vi "Make Joystick JSON.vi"(9 "Force":bool, 10 "Joystick prev":T1={"type"="Joystick", "device"="3", "name"="", "data"={"<init"=FALSE, ">buttons"=[], ">povs"=[], ">axes"=[], "<left_rumble"=0.0, "<right_rumble"=0.0, "<outputs"=0}}, 11 "Joystick new":T1={"type"="Joystick", "device"="3", "name"="", "data"={"<init"=FALSE, ">buttons"=[], ">povs"=[], ">axes"=[], "<left_rumble"=0.0, "<right_rumble"=0.0, "<outputs"=0}}) -> (3 "JSON delta":string)   [LabVIEW 2019]
uses:
  Joystick data proto.ctl
  Joystick proto.ctl
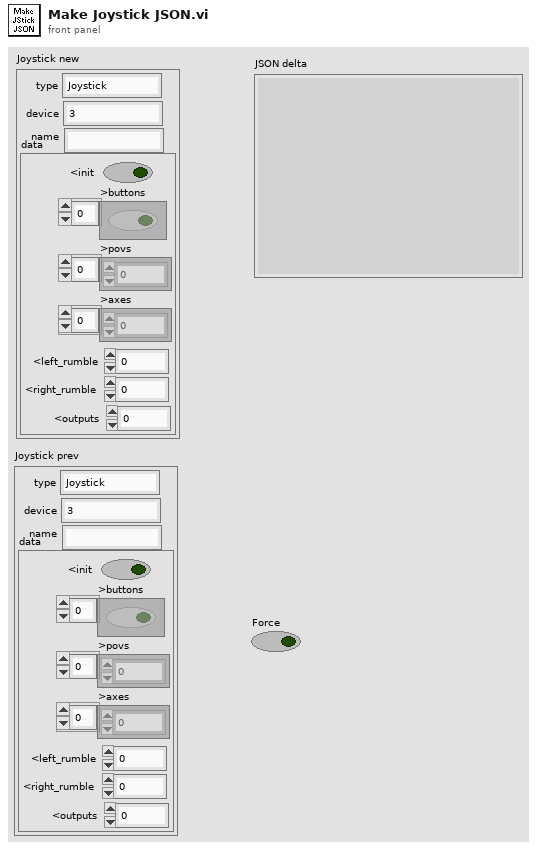
[diagram p1: front panel]
types:
  T1 = typedef "Joystick proto.ctl" = cluster{"type":string, "device":string, "name":string, "data":T2}
  T2 = typedef "Joystick data proto.ctl" = cluster{"<init":bool, ">buttons":bool[], ">povs":i32[], ">axes":i32[], "<left_rumble":dbl, "<right_rumble":dbl, "<outputs":i32}
  T3 = cluster{"type":bool, "device":bool, "name":bool, "data":cluster{"<init":bool, ">buttons":bool[], ">povs":bool[], ">axes":bool[], "<left_rumble":bool, "<right_rumble":bool, "<outputs":bool}}
  T4 = cluster{"<init":bool, ">buttons":bool[], ">povs":bool[], ">axes":bool[], "<left_rumble":bool, "<right_rumble":bool, "<outputs":bool}
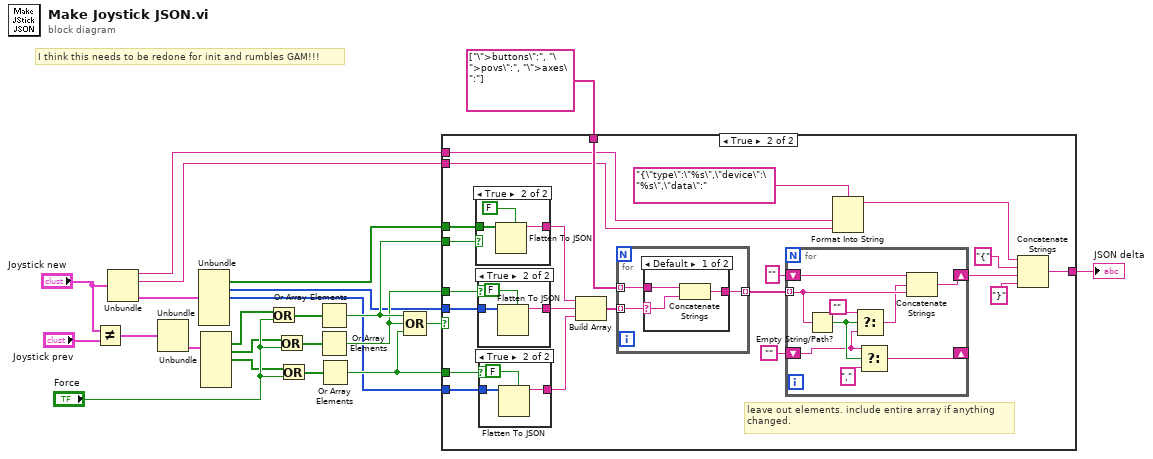
[diagram p0: block diagram]
diagram:
  # "I think this needs to be redone for init and rumbles GAM!!!"
  n1 = Not Equal?(x="Joystick new", y="Joystick prev") -> (x != y?=w7:T3)
  n2 = Unbundle("Joystick new") -> ("type"=w14:string, "device"=w15:string, "data"=w13:T2)  [unwired: 1 out]
  n3 = Unbundle(w7) -> ("data"=w12:T4)  [unwired: 3 out]
  n4 = Unbundle(w13) -> (">buttons"=w4:bool[], ">povs"=w5:i32[], ">axes"=w6:i32[])  [unwired: 4 out]
  n5 = Unbundle(w12) -> (">buttons"=w1:bool[], ">povs"=w2:bool[], ">axes"=w3:bool[])  [unwired: 4 out]
  n6 = Or(x=w1, y="Force") -> (x .or. y?=w10:bool[])
  n7 = Or(x=w2, y="Force") -> (x .or. y?=w9:bool[])
  n8 = Or(x=w3, y="Force") -> (x .or. y?=w8:bool[])
  n9 = Or Array Elements(Boolean array=w10) -> (logical OR=w19:bool)
  n10 = Or Array Elements(Boolean array=w9) -> (logical OR=w18:bool)
  n11 = Or Array Elements(Boolean array=w8) -> (logical OR=w17:bool)
  n12 = Compound Arithmetic op=OR(w19, w18, w17) -> (w16:bool)
  n13 = case shown="True" w16 {
    tunnel: w19 -> [_ w45]
    tunnel: w4 -> [_ w44]
    tunnel: w18 -> [_ w43]
    tunnel: w5 -> [_ w42]
    tunnel: w17 -> [_ w41]
    tunnel: w6 -> [_ w40]
    tunnel: string[] ["\">buttons\":", "\">povs\":", "\">axes\":"] -> [_ w36]
    tunnel: [_ w30] -> w20
    tunnel: w15 -> [_ w25]
    tunnel: w14 -> [_ w24]
    frame False {
    }
    frame True {
      # "leave out elements. include entire array if anything\nchanged."
      n14 = case shown="True" w45 {
        tunnel: w44 -> [_ w69]
        tunnel: [_ w67] -> w39
        frame False {
        }
        frame True {
          n15 = Flatten To JSON(enable LabVIEW extensions? (T)=FALSE, anything=w69) -> (JSON string=w67:string)  [unwired: 1 in, 1 out]
        }
      }
      n16 = case shown="True" w43 {
        tunnel: w42 -> [_ w66]
        tunnel: [_ w64] -> w38
        frame False {
        }
        frame True {
          n17 = Flatten To JSON(enable LabVIEW extensions? (T)=FALSE, anything=w66) -> (JSON string=w64:string)  [unwired: 1 in, 1 out]
        }
      }
      n18 = case shown="True" w41 {
        tunnel: w40 -> [_ w63]
        tunnel: [_ w61] -> w37
        frame False {
        }
        frame True {
          n19 = Flatten To JSON(enable LabVIEW extensions? (T)=FALSE, anything=w63) -> (JSON string=w61:string)  [unwired: 1 in, 1 out]
        }
      }
      n20 = Build Array(w39, w38, w37) -> (w35:string[])
      n21 = for {
        tunnel: w36 -> [w56] mode=indexing
        tunnel: w35 -> [w57] mode=indexing
        tunnel: [w55] -> w34 mode=indexing
        n22 = case shown="Default" w57 {
          selector: w57 -> [w59 _]
          tunnel: w56 -> [w60 _]
          tunnel: [w58 _] -> w55
          frame Default {
            n23 = Concatenate Strings(w60, w59) -> (w58:string)
          }
          frame "" {
          }
        }
      }
      n24 = for {
        tunnel: w34 -> [w51] mode=indexing
        shift-right: [w52] -> w33
        shift-left: "" -> [w54]
        shift-right: [w50] -> _
        shift-left: "" -> [w46]
        n25 = Empty String/Path?(string/path=w51) -> (empty?=w49:bool)
        n26 = Select(t="", s=w49, f=w46) -> (s? t:f=w48:string)
        n27 = Select(t=w46, s=w49, f=",") -> (s? t:f=w50:string)
        n28 = Concatenate Strings(w54, w48, w51) -> (w52:string)
      }
      n29 = Format Into String(format string="{\"type\":\"%s\",\"device\":\"%s\",\"data\":", w24, w25) -> (resulting string=w26:string)  [unwired: 2 in, 1 out]
      n30 = Concatenate Strings(w26, "{", w33, "}") -> (w30:string)
    }
  }
  "JSON delta" <- w20
